vi "Loopbadk Test.vi"() -> ()   [LabVIEW 2009]
uses:
  <vilib>/Instr/_visa.llb/VISA Configure Serial Port (Instr).vi
panel:
  out "error out":errorcluster
  in  "Enable Termination\nChar (T)":bool
  in  "termination char\n(0xA = '\\n' = LF)":u8=10 format="%.0x"
  in  "flow control (0:none)":u16(ring) items=["None", "XON/XOFF", "RTS/CTS", "XON/XOFF & RTS/CTS", "DTR/DSR", "XON/XOFF & DTR/DSR"]
  in  "stop bits (10: 1 bit)":u16(ring)=10 items=["1.0"=10, "1.5"=15, "2.0"=20]
  in  "parity (0:none)":enum16{"None", "Odd", "Even", "Mark", "Space"}(ring)
  in  "data bits (8)":u16=8 min=5 max=8 step=1
  in  "baud rate (9600)":u32=19200
  in  "VISA resource name":refnum<visa-resource-name>="COM24"
  in  "timeout (10sec)":u32=120
  out "x = y?":bool
  in  "TestArray":u8[](array[numeric])=[10, 11, 12, 13] format="%02x"
  in  "Stop":bool
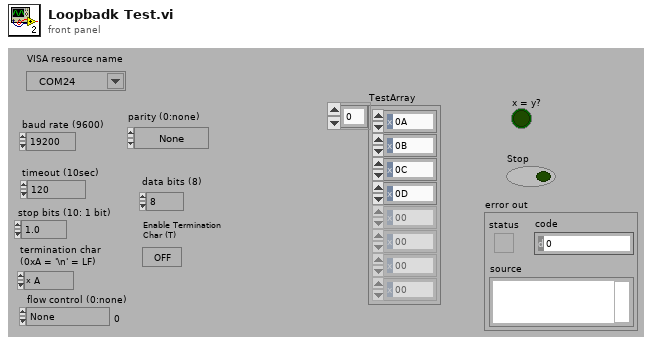
[diagram p1: front panel]
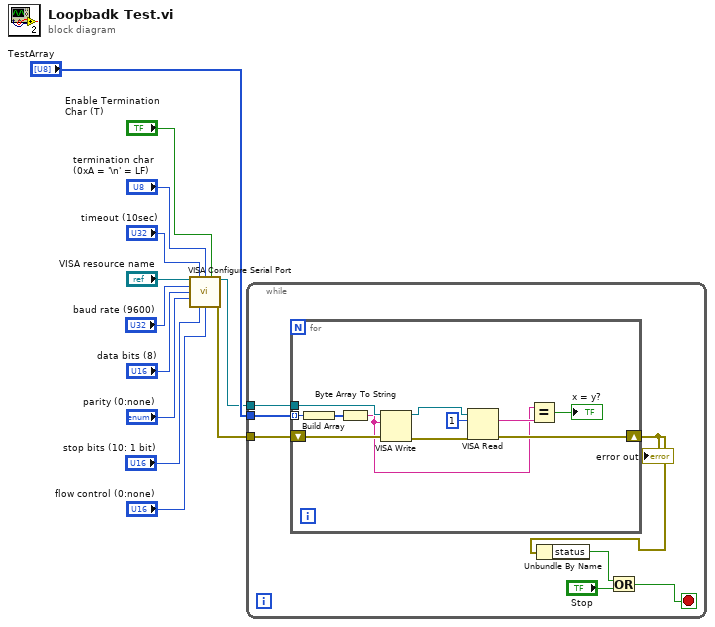
[diagram p0: block diagram]
diagram:
  n1 = call-poly "VISA Configure Serial Port"("VISA resource name"="VISA resource name", "timeout (10sec)"="timeout (10sec)", "termination char\n(0xA = '\\n' = LF)"="termination char\n(0xA = '\\n' = LF)", "Enable Termination\nChar (T)"="Enable Termination\nChar (T)", "baud rate (9600)"="baud rate (9600)", "data bits (8)"="data bits (8)", "parity (0:none)"="parity (0:none)", "stop bits (10: 1 bit)"="stop bits (10: 1 bit)", "flow control (0:none)"="flow control (0:none)") -> ("VISA resource name out"=w10:refnum<visa-resource-name>, "error out"=w11:errorcluster)  [unwired: 5 in]
  n2 = while {
    tunnel: "TestArray" -> [w17]
    tunnel: w11 -> [w14]
    tunnel: w10 -> [w13]
    stop <- w19 stop-if-true
    n3 = for {
      tunnel: w17 -> [w30] mode=indexing
      shift-right: [w26] -> w15
      shift-left: w14 -> [w25]
      tunnel: w13 -> [w24]
      n4 = Build Array(w30) -> (w29:u8[])
      n5 = Byte Array To String(unsigned byte array=w29) -> (string=w21:string)
      n6 = VISA Write(VISA resource name=w24, write buffer=w21, error in (no error)=w25) -> (VISA resource name out=w23:refnum<visa-resource-name>, error out=w27:errorcluster)  [unwired: 1 out]
      n7 = VISA Read(VISA resource name=w23, byte count=u32 1, error in (no error)=w27) -> (read buffer=w22:string, error out=w26:errorcluster)  [unwired: 2 out]
      n8 = Equal?(x=w21, y=w22) -> (x = y?=→"x = y?":bool)
    }
    "error out" <- w15
    n9 = Unbundle By Name(w15) -> ("status"=w16:bool)
    n10 = Or(x=w16, y="Stop") -> (x .or. y?=w19:bool)
  }
